vi "Write Timeout.vi"(8 "error in (no error)":errorcluster, 10 "timeout (ms) [500]":i32=500, 11 "RemoteControl in":refnum<class "RemoteControl.lvclass">) -> (0 "error out":errorcluster, 3 "RemoteControl out":refnum<class "RemoteControl.lvclass">)   [LabVIEW 2019, in "RemoteControl.lvlib" / "RemoteControl.lvclass"]
uses:
  RemoteControl.lvclass
  RemoteControl.lvclass/RemoteControl.ctl
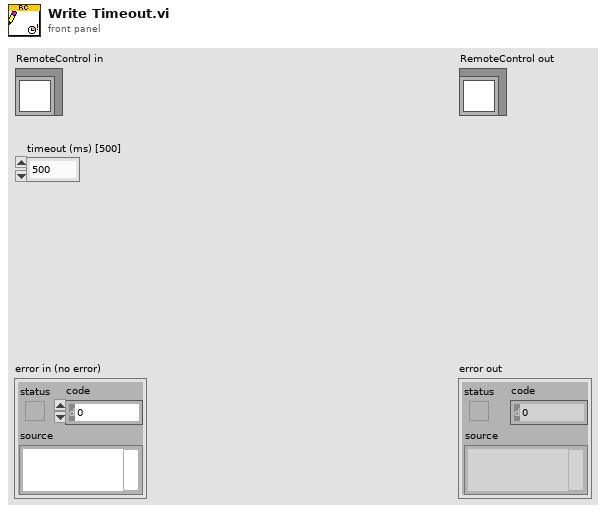
[diagram p1: front panel]
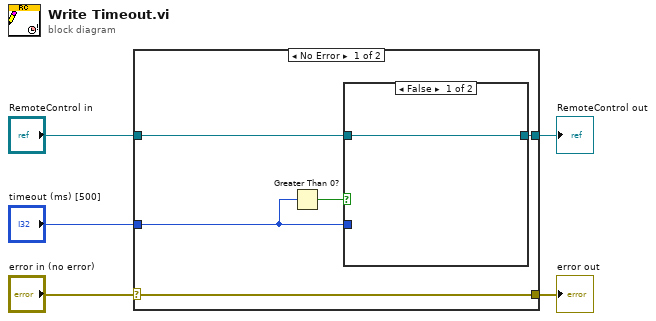
[diagram p0: block diagram]
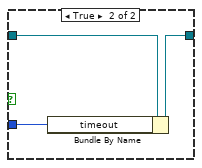
[diagram p2: hidden frame]
diagram:
  n1 = case shown="No Error" "error in (no error)" {
    selector: "error in (no error)" -> [w10 w15]
    tunnel: [w10 w15] -> w4
    tunnel: [w8 w16] -> w2
    tunnel: "RemoteControl in" -> [w9 w16]
    tunnel: "timeout (ms) [500]" -> [w7 _]
    frame No Error {
      n2 = Greater Than 0?(x=w7) -> (x > 0?=w6:bool)
      n3 = case shown="False" w6 {
        tunnel: w9 -> [w11 w14]
        tunnel: [w11 w13] -> w8
        tunnel: w7 -> [_ w12]
        frame False {
        }
        frame True {
          n4 = Bundle By Name(cluster=w14, "timeout"=w12) -> (w13:refnum<class "RemoteControl.lvclass">)
        }
      }
    }
    frame Error {
    }
  }
  "error out" <- w4
  "RemoteControl out" <- w2
